vi "Defaults-saved-subvi.vi"() -> ()   [LabVIEW 2014]
uses:
  Start all VIs Globals.vi
panel:
  in  "error in (no error)":errorcluster
  out "error out":errorcluster
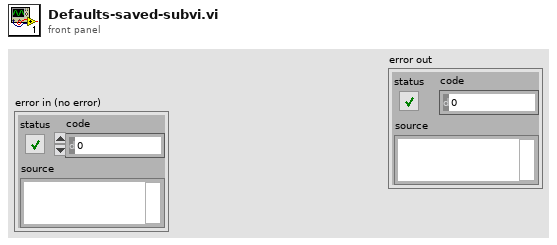
[diagram p1: front panel]
types:
  T1 = cluster{"Shutter Control":path, "Stage Control":path, "Camera & Acquisition VIs":path, "TIRF Lock":path}
  T2 = enum32{"Invalid", "Standard", "Closed", "Hidden", "Minimized", "Maximized"}
  T3 = enum32{"Bad", "Idle", "Run top level", "Running"}
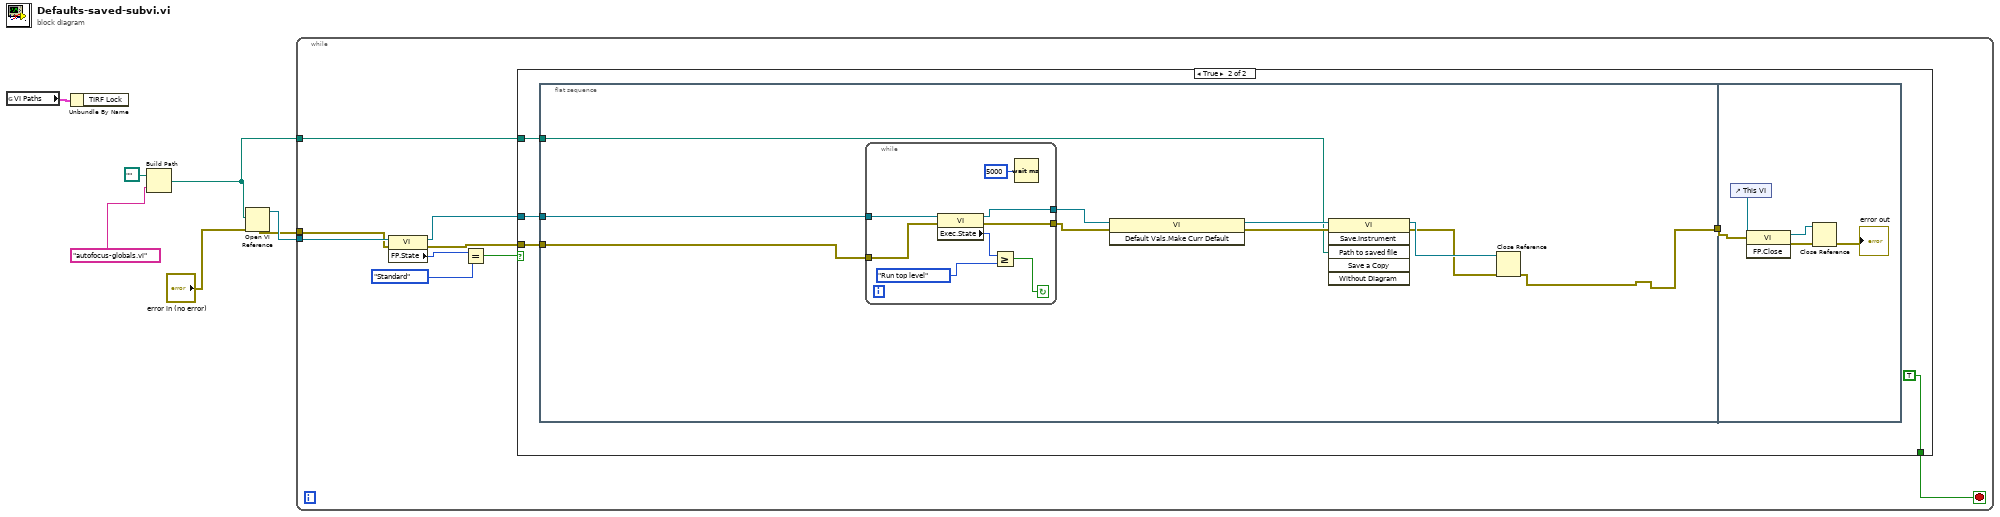
[diagram p0: block diagram]
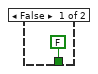
[diagram p2: hidden frame]
diagram:
  n1 = global read "Start all VIs Globals.vi" "VI Paths"() -> (w6:T1)
  n2 = Unbundle By Name(w6) -> ()  [unwired: 1 out]
  n3 = Build Path(base path=path "", name or relative path="autofocus-globals.vi") -> (appended path=w2:path)
  n4 = Open VI Reference(vi path=w2, error in (no error)="error in (no error)") -> (vi reference=w5:refnum<vi>, error out=w4:errorcluster)  [unwired: 4 out]
  n5 = while {
    tunnel: w5 -> [w14]
    tunnel: w4 -> [w13]
    tunnel: w2 -> [w8]
    stop <- w10 stop-if-true
    n6 = property class="VI"(reference=w14, error in=w13) -> (reference out=w11:refnum<vi>, error out=w12:errorcluster, "FP.State"=w16:T2)
    n7 = Equal?(x=w16, y=T2."Standard") -> (x = y?=w15:bool)
    n8 = case shown="True" w15 {
      tunnel: w12 -> [_ w21]
      tunnel: w11 -> [_ w20]
      tunnel: [FALSE TRUE] -> w10
      tunnel: w8 -> [_ w18]
      frame False {
      }
      frame True {
        n9 = flat-sequence {
          tunnel: [w23] -> w22
          tunnel: w21 -> [w27]
          tunnel: w20 -> [w26]
          tunnel: w18 -> [w24]
          tunnel: w22 -> [w44]
          frame #0 {
            n10 = while {
              tunnel: w26 -> [w39]
              tunnel: w27 -> [w38]
              tunnel: [w34] -> w32
              tunnel: [w33] -> w31
              stop <- w35 continue-if-true
              n11 = property class="VI"(reference=w39, error in=w38) -> (reference out=w34:refnum<vi>, error out=w33:errorcluster, "Exec.State"=w36:T3)
              n12 = Greater Or Equal?(x=w36, y=T3."Run top level" ("Execution:State")) -> (x >= y?=w35:bool)
              n13 = Wait (ms)(milliseconds to wait=u32 5000) -> ()  [unwired: 1 out]
            }
            n14 = invoke class="VI" method="Default Vals.Make Curr Default"(reference=w32, error in=w31) -> (reference out=w25:refnum<vi>, error out=w30:errorcluster)  [unwired: 1 in, 1 out]
            n15 = invoke class="VI" method="Save.Instrument"(reference=w25, error in=w30, "Path to saved file"=w24) -> (reference out=w29:refnum<vi>, error out=w28:errorcluster)  [unwired: 3 in, 4 out]
            n16 = Close Reference(reference=w29, error in (no error)=w28) -> (error out=w23:errorcluster)
          }
          frame #1 {
            n17 = control-ref of="This VI"() -> (w45:refnum<vi>)
            n18 = invoke class="VI" method="FP.Close"(reference=w45, error in=w44) -> (reference out=w43:refnum<vi>, error out=w42:errorcluster)  [unwired: 1 in, 1 out]
            n19 = Close Reference(reference=w43, error in (no error)=w42) -> (error out=→"error out":errorcluster)
          }
        }
      }
    }
  }
